vi "Get NVMEM Bytes.vi"(0 "SLSC Remote In":refnum<class "SLSC Remote.lvclass">, 5 "NVMEM area":refnum<k21>="$DefaultNVMEMAreas", 7 "data address":u32 format="%.0x", 9 "data size":u32, 11 "error in (no error)":errorcluster) -> (4 "SLSC Remote Out":refnum<class "SLSC Remote.lvclass">, 6 "NVMEM area out":refnum<k21>, 8 "next data address":u32 format="%.0x", 10 "data out":u8[](array[numeric]) format="%.0x", 15 "error out":errorcluster)   [LabVIEW 2015, in "SLSC Remote.lvclass"]
uses:
  SLSC Remote.lvclass
  <vilib>/NI/i3 JSON/JSON Generation/Create Value Files/Create Value - Object.vi
  <vilib>/NI/i3 JSON/JSON Generation/Add Object Parameter Files/Add Object Parameter - String.vi
  <vilib>/NI/i3 JSON/JSON Generation/Add Object Parameter Files/Add Object Parameter - Numeric.vi
  <vilib>/NI/NI JSONRPC Server Framework/Classes/Server/Format Client Request (Auto-Increment).vi
  <vilib>/httpClient/POSTBuffer.vi
  <vilib>/NI/i3 JSON/JSON Parsing/Get Object Parameter Files/Get Object Parameter - Numeric.vi
  <vilib>/NI/i3 JSON/JSON Parsing/Get Object Parameter Files/Get Object Parameter - 1D Array Double.vi
  <vilib>/NI/NI JSONRPC Server Framework/Classes/Server/JSONRPC Server.lvclass
  <vilib>/NI/i3 JSON/i3-json.lvlib
  <vilib>/httpClient/LabVIEWHTTPClient.lvlib
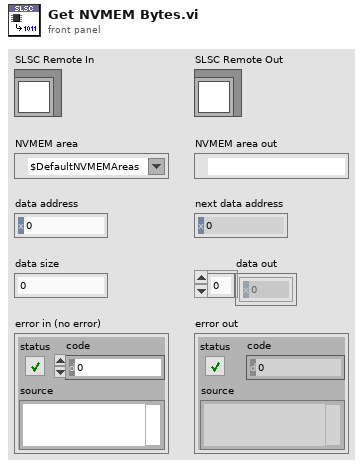
[diagram p1: front panel]
types:
  T1 = typedef "LabVIEWHTTPClient.lvlib/ClientHandle.ctl" = refnum<k1>
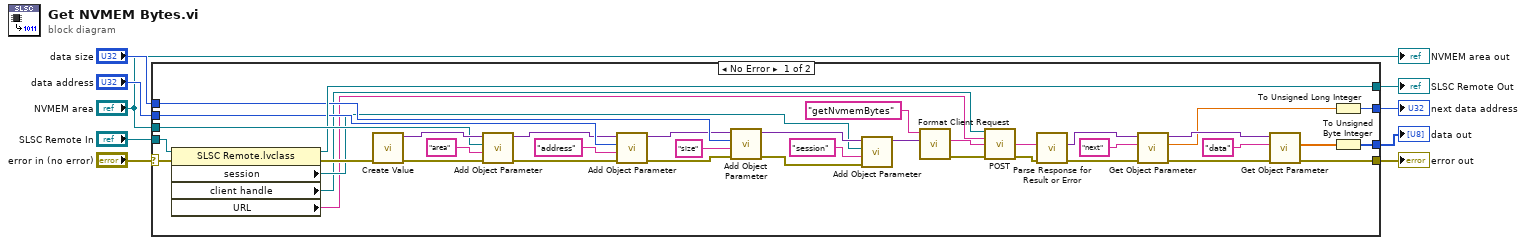
[diagram p0: block diagram]
diagram:
  n1 = case shown="No Error" "error in (no error)" {
    selector: "error in (no error)" -> [w42 w50]
    tunnel: "NVMEM area" -> [w47 _]
    tunnel: [w45 w49] -> w6
    tunnel: "data address" -> [w43 _]
    tunnel: "data size" -> [w38 _]
    tunnel: [w14 w50] -> w4
    tunnel: "SLSC Remote In" -> [w21 w49]
    tunnel: [w10 _] -> w2
    tunnel: [w12 _] -> w1
    frame No Error {
      n2 = property class="SLSC Remote.lvclass"(reference=w21, error in=w42) -> (reference out=w45:refnum<class "SLSC Remote.lvclass">, error out=w41:errorcluster, "session"=w30:refnum<k21>, "client handle"=w28:T1, "URL"=w27:string)
      n3 = call-poly <vilib>:"Create Value.vi"("error in (no error)"=w41) -> ("error out"=w40:errorcluster, "JSON Tree"=w48:variant)  [unwired: 9 in]
      n4 = call-poly <vilib>:"Add Object Parameter.vi"("error in (no error)"=w40, "Name"="area", "String"=w47, "JSON Tree in (JSON Object)"=w48) -> ("error out"=w39:errorcluster, "JSON Tree out (JSON Object)"=w35:variant)  [unwired: 6 in]
      n5 = call-poly <vilib>:"Add Object Parameter.vi"("error in (no error)"=w39, "Name"="address", "Numeric"=w43, "JSON Tree in (JSON Object)"=w35) -> ("error out"=w33:errorcluster, "JSON Tree out (JSON Object)"=w34:variant)  [unwired: 6 in]
      n6 = call-poly <vilib>:"Add Object Parameter.vi"("error in (no error)"=w33, "Name"="size" ("String"), "Numeric"=w38, "JSON Tree in (JSON Object)"=w34) -> ("error out"=w31:errorcluster, "JSON Tree out (JSON Object)"=w32:variant)  [unwired: 6 in]
      n7 = call-poly <vilib>:"Add Object Parameter.vi"("error in (no error)"=w31, "Name"="session", "String"=w30, "JSON Tree in (JSON Object)"=w32) -> ("JSON Tree out (JSON Object)"=w22:variant)  [unwired: 6 in, 1 out]
      n8 = call-poly <vilib>:"Format Client Request.vi"("params"=w22, "method"="getNvmemBytes") -> ("error out"=w26:errorcluster, "Request String"=w36:string)  [unwired: 8 in]
      n9 = call-poly <vilib>:"POST.vi"("client handle"=w28, "url"=w27, "buffer"=w36, "error in (no error)"=w26) -> ("body"=w24:string, "error out"=w23:errorcluster)  [unwired: 8 in, 2 out]
      n10 = call <vilib>:"Parse Response for Result or Error.vi"("error in"=w23, "Response String In"=w24) -> ("error out"=w18:errorcluster, "Result or Error Data"=w20:variant)  [unwired: 7 in, 1 out]
      n11 = call-poly <vilib>:"Get Object Parameter.vi"("error in (no error)"=w18, "Parameter Name"="next", "JSON Tree In (JSON Object)"=w20) -> ("error out"=w15:errorcluster, "Double Value"=w13:dbl, "JSON Tree Out Passthrough"=w17:variant)  [unwired: 5 in, 1 out]
      n12 = call-poly <vilib>:"Get Object Parameter.vi"("error in (no error)"=w15, "Parameter Name"="data", "JSON Tree In (JSON Object)"=w17) -> ("error out"=w14:errorcluster, "1D Double Array Value"=w11:dbl[])  [unwired: 5 in, 2 out]
      n13 = To Unsigned Long Integer(number=w13) -> (unsigned 32bit integer=w12:u32)
      n14 = To Unsigned Byte Integer(number=w11) -> (unsigned 8bit integer=w10:u8[])
    }
    frame Error {
    }
  }
  "error out" <- w4
  "data out" <- w2
  "next data address" <- w1
  "SLSC Remote Out" <- w6
  "NVMEM area out" <- "NVMEM area"
